vi "Write objectiveVector.vi"(8 "error in (no error)":errorcluster, 10 "objectiveVector":T1[](array[typedef]), 11 "Evaluator in":refnum<class "Evaluator.lvclass">) -> (0 "error out":errorcluster, 3 "Evaluator out":refnum<class "Evaluator.lvclass">)   [LabVIEW 2023, in "Evaluator.lvclass"]
uses:
  Evaluator.lvclass
  Objectives.ctl
  Evaluator.lvclass/Evaluator.ctl
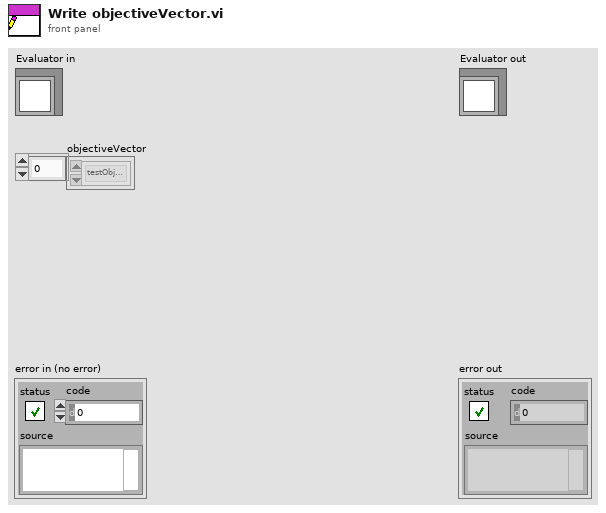
[diagram p1: front panel]
types:
  T1 = typedef "Evaluator.lvclass/Objectives.ctl" = enum16{"testObjective"}
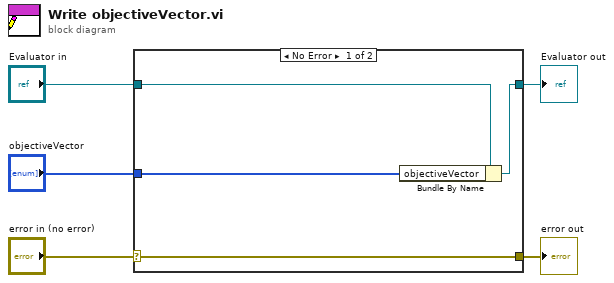
[diagram p0: block diagram]
diagram:
  n1 = case shown="No Error" "error in (no error)" {
    selector: "error in (no error)" -> [w9 w10]
    tunnel: [w9 w10] -> w4
    tunnel: [w7 w11] -> w2
    tunnel: "Evaluator in" -> [w8 w11]
    tunnel: "objectiveVector" -> [w6 _]
    frame No Error {
      n2 = Bundle By Name(cluster=w8, "objectiveVector"=w6) -> (w7:refnum<class "Evaluator.lvclass">)
    }
    frame Error {
    }
  }
  "error out" <- w4
  "Evaluator out" <- w2
